vi "MFP3D Driver.vi"() -> ()   [LabVIEW 2019]
uses:
  <userlib>/LevyLab/Relay Box/Typedefs/Resistor--enum.ctl
  subVIs/Driver Variables_MFP3D.vi
  subVIs/Global Variables.vi
  <userlib>/LevyLab/Relay Box/Relay-Box.lvclass
panel:
  out "Boolean":bool
  in  "Data Queue":refnum<queue>
  in  "Amplifier Setting":dbl=-15.0
  in  "Interpolation Distance (µm)":dbl=0.1
  in  "Background Image":refnum<vi>
  in  "Inkscape File (.svg)":refnum<vi>
  in  "Run":refnum<vi>
  in  "Abort":refnum<vi>
  in  "Lithography Data":T2(array[cluster])
  in  "Display Wave":bool
  in  "PID Close":bool
  in  "Withdraw Tip When Done":bool=TRUE
  in  "Move Z Set Point":dbl=-1.3
  in  "Z Set Point":dbl=-0.05
  # "MFP3D Driver"
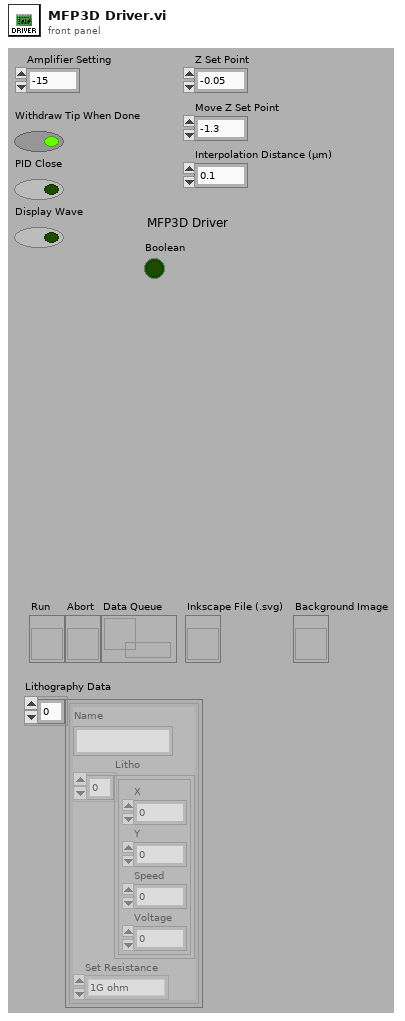
[diagram p1: front panel]
types:
  T1 = typedef "Relay-Box.lvclass/Resistor--enum.ctl" = enum16{"open", "discharge tip", "0 ohms", "100k ohm", "10M ohm", "1G ohm"}
  T2 = cluster{"Name":string, "Litho":cluster{"X":dbl, "Y":dbl, "Speed":dbl, "Voltage":dbl}[], "Set Resistance":T1}[]
  T3 = cluster{"Coordinate":cluster{"X":dbl, "Y":dbl}, "Speed":dbl, "Voltage":dbl, "RGB Value":dbl, "Name":string, "Set Resistance":T1}[][]
  T4 = cluster{"Array":cluster{"Coordinate":cluster{"X":dbl, "Y":dbl}, "Speed":dbl, "Voltage":dbl, "RGB Value":dbl, "Name":string, "Set Resistance":T1}[][], "Size":cluster{"Width":dbl, "Height":dbl}, cluster{"X Offset":dbl, "Y Offset":dbl}, "Interpolation Distance (µm)":dbl, "Z Set Point":dbl, "Move Z Set Point":dbl, "PID Close":bool, "Display Wave":bool, "Run":refnum<vi>}
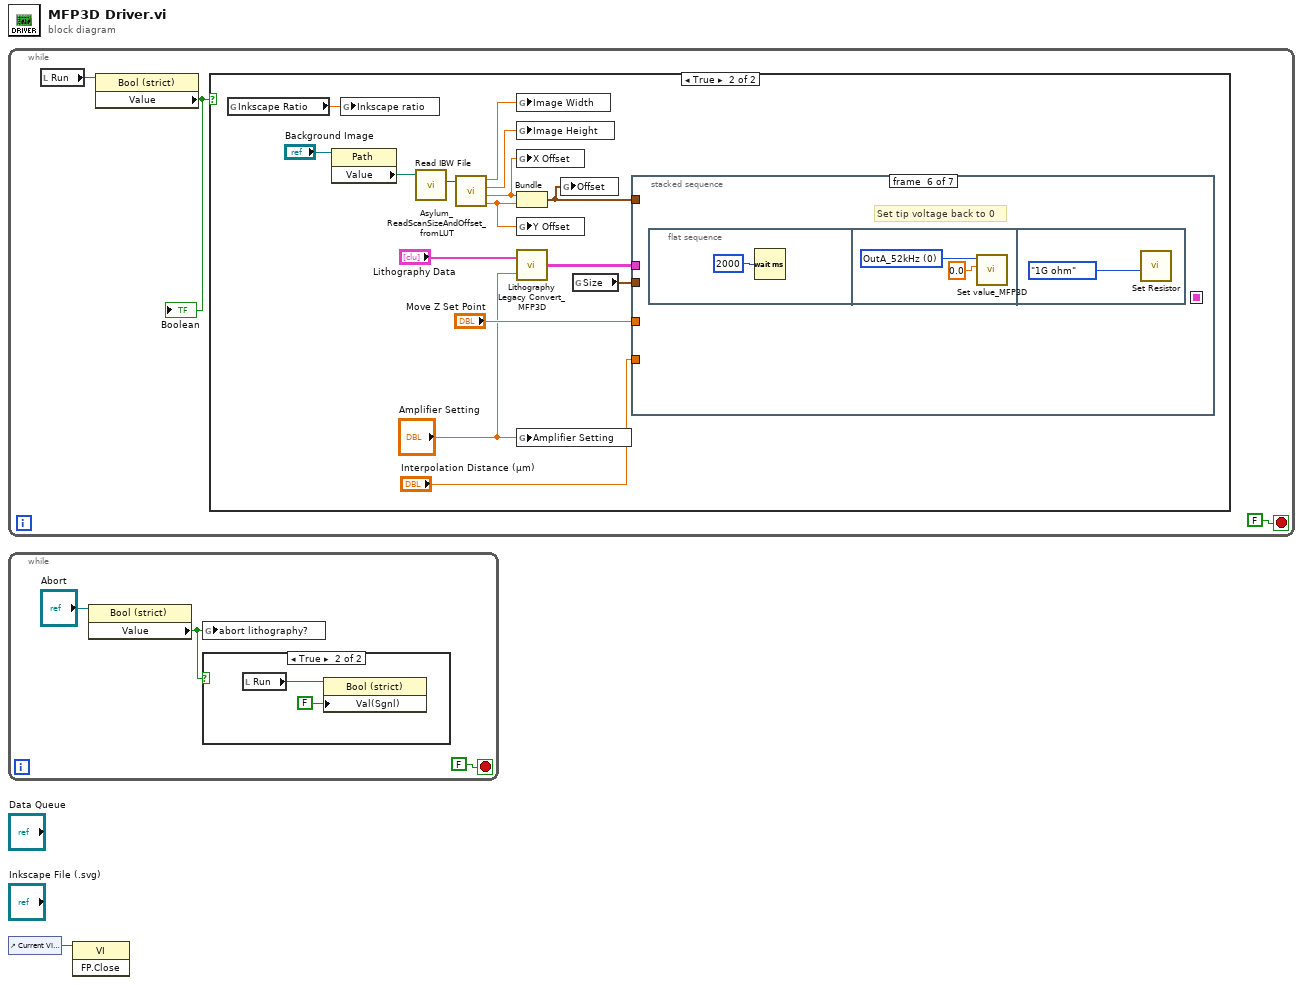
[diagram p0: block diagram]
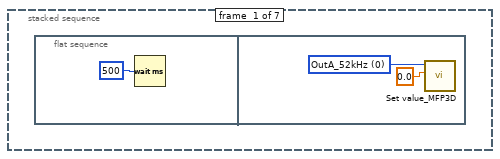
[diagram p3: hidden frame]
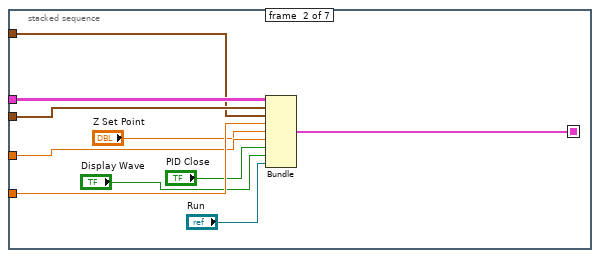
[diagram p4: hidden frame]
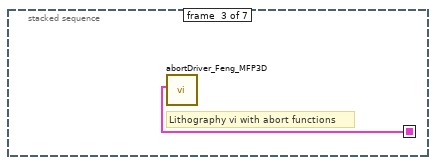
[diagram p5: hidden frame]
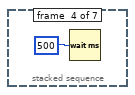
[diagram p6: hidden frame]
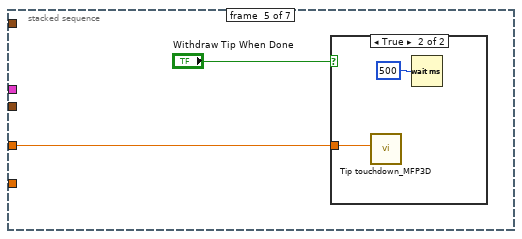
[diagram p7: hidden frame]
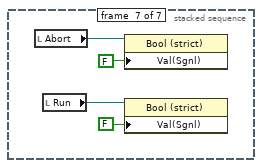
[diagram p9: hidden frame]
diagram:
  n1 = while {
    stop <- FALSE stop-if-true
    n2 = local read "Run"() -> (w3:refnum<vi>)
    n3 = property class="Bool (strict)"(reference=w3) -> ("Value"=w2:bool)  [unwired: 1 in, 2 out]
    "Boolean" <- w2
    n4 = case shown="True" w2 {
      frame False {
      }
      frame True {
        n5 = global read "Global Variables.vi" "Inkscape Ratio"() -> (w14:dbl)
        n6 = property class="Path"(reference="Background Image") -> ("Value"=w9:path)  [unwired: 1 in, 2 out]
        n7 = global write "Driver Variables_MFP3D.vi" "Inkscape ratio"(w14) -> ()
        n8 = call "Read IBW File.vi"("Path"=w9) -> ("Notes LUT"=w10:variant)  [unwired: 8 in, 2 out]
        n9 = call "Asylum_ReadScanSizeAndOffset_fromLUT.vi"("Notes LUT"=w10) -> ("Y Offset"=w5:dbl, "X Offset"=w6:dbl, "Y Range"=w7:dbl, "X Range"=w8:dbl)  [unwired: 7 in]
        n10 = global write "Driver Variables_MFP3D.vi" "Image Width"(w8) -> ()
        n11 = global write "Driver Variables_MFP3D.vi" "Image Height"(w7) -> ()
        n12 = global write "Driver Variables_MFP3D.vi" "X Offset"(w6) -> ()
        n13 = Bundle("X Offset"=w6, "Y Offset"=w5) -> (w15:cluster{"X Offset":dbl, "Y Offset":dbl})  [unwired: 1 in]
        n14 = global write "Driver Variables_MFP3D.vi" "Y Offset"(w5) -> ()
        n15 = call "Lithography Legacy Convert_MFP3D.vi"("Amplifier Setting"="Amplifier Setting", "Lithography Data"="Lithography Data") -> ("Array"=w13:T3)
        n16 = global write "Driver Variables_MFP3D.vi" "Amplifier Setting"("Amplifier Setting") -> ()
        n17 = global write "Global Variables.vi" "Offset"(w15) -> ()
        n18 = global read "Global Variables.vi" "Size"() -> (w18:cluster{"Width":dbl, "Height":dbl})
        n19 = stacked-sequence {
          seq-local: [_ w27 _ _ _ _ _] -> [_ _ w33 _ _ _ _]
          tunnel: w13 -> [_ w32 _ _ _ _ _]
          tunnel: w18 -> [_ w31 _ _ _ _ _]
          tunnel: "Interpolation Distance (µm)" -> [_ w29 _ _ _ _ _]
          tunnel: w15 -> [_ w30 _ _ _ _ _]
          tunnel: "Move Z Set Point" -> [_ w28 _ _ w36 _ _]
          frame #0 {
            n20 = flat-sequence {
              frame #0 {
                n21 = Wait (ms)(milliseconds to wait=u32 500) -> ()  [unwired: 1 out]
              }
              frame #1 {
                w22 = u16 0 items=["OutA_52kHz", "OutB_52kHz", "OutC_78Hz", "PiezoX", "PiezoY", "PiezoZ", "DDS_Frequency1", "DDS_Frequency2", "DDS_Amplitude1", "DDS_Amplitude2", "DDS_DCOffset", "\"Setpoint%PIDSLoop.3\"", "\"Setpoint%PIDSLoop.4\"", ""] ("Output")
                n22 = call "Set value_MFP3D.vi"("Value"=0.0, "Output"=w22) -> ()  [unwired: 9 in, 1 out]
              }
            }
          }
          frame #1 {
            n23 = Bundle("Array"=w32, "Size"=w31, w30, "Interpolation Distance (µm)"=w29, "Z Set Point"="Z Set Point", "Move Z Set Point"=w28, "PID Close"="PID Close", "Display Wave"="Display Wave", "Run"="Run") -> (w27:T4)  [unwired: 1 in]
          }
          frame #2 {
            # "Lithography vi with abort functions"
            n24 = call "abortDriver_Feng_MFP3D.vi"("litho comm"=w33) -> ()  [unwired: 11 in]
          }
          frame #3 {
            n25 = Wait (ms)(milliseconds to wait=u32 500) -> ()  [unwired: 1 out]
          }
          frame #4 {
            n26 = case shown="True" "Withdraw Tip When Done" {
              tunnel: w36 -> [_ w37]
              frame False {
              }
              frame True {
                n27 = call "Tip touchdown_MFP3D.vi"("Z SetPoint"=w37) -> ()  [unwired: 11 out]
                n28 = Wait (ms)(milliseconds to wait=u32 500) -> ()  [unwired: 1 out]
              }
            }
          }
          frame #5 {
            # "Set tip voltage back to 0"
            n29 = flat-sequence {
              frame #0 {
                n30 = Wait (ms)(milliseconds to wait=u32 2000) -> ()  [unwired: 1 out]
              }
              frame #1 {
                w41 = u16 0 items=["OutA_52kHz", "OutB_52kHz", "OutC_78Hz", "PiezoX", "PiezoY", "PiezoZ", "DDS_Frequency1", "DDS_Frequency2", "DDS_Amplitude1", "DDS_Amplitude2", "DDS_DCOffset", "\"Setpoint%PIDSLoop.3\"", "\"Setpoint%PIDSLoop.4\"", ""] ("Output")
                n31 = call "Set value_MFP3D.vi"("Value"=0.0, "Output"=w41) -> ()  [unwired: 9 in, 1 out]
              }
              frame #2 {
                n32 = call <userlib>:"Set Resistor.vi"("Set Resistance"=Resistor--enum."1G ohm") -> ()  [unwired: 10 in, 1 out]
              }
            }
          }
          frame #6 {
            n33 = local read "Abort"() -> (w43:refnum<vi>)
            n34 = local read "Run"() -> (w46:refnum<vi>)
            n35 = property class="Bool (strict)"(reference=w43, "Val(Sgnl)"=FALSE ("Value (Signaling)")) -> ()  [unwired: 1 in, 2 out]
            n36 = property class="Bool (strict)"(reference=w46, "Val(Sgnl)"=FALSE ("Value (Signaling)")) -> ()  [unwired: 1 in, 2 out]
          }
        }
      }
    }
  }
  n37 = while {
    stop <- FALSE stop-if-true
    n38 = property class="Bool (strict)"(reference="Abort") -> ("Value"=w47:bool)  [unwired: 1 in, 2 out]
    n39 = global write "Driver Variables_MFP3D.vi" "abort lithography?"(w47) -> ()
    n40 = case shown="True" w47 {
      frame False {
      }
      frame True {
        n41 = local read "Run"() -> (w51:refnum<vi>)
        n42 = property class="Bool (strict)"(reference=w51, "Val(Sgnl)"=FALSE ("Value (Signaling)")) -> ()  [unwired: 1 in, 2 out]
      }
    }
  }
  n43 = control-ref of="Current VI Reference"() -> (w1:refnum<vi>)
  n44 = invoke class="VI" method="FP.Close"(reference=w1) -> ()  [unwired: 2 in, 3 out]
